vi "_Read.vi"(8 "error in (no error)":errorcluster, 11 "Readable in":refnum<class "Readable.lvclass">) -> (0 "error out":errorcluster, 2 "Data Points":T1, 3 "Readable out":refnum<class "Readable.lvclass">)   [LabVIEW 2009, in "Readable.lvclass"]
doc: "(Protected, Dynamic, Pure Virtual/Abstract) Perform a measurement and return one or more channels of data. Outsiders should not call this method, but instead the public \"Read Data.vi\"."
uses:
  Readable.lvclass
  Data Points.ctl
  Data Point.ctl
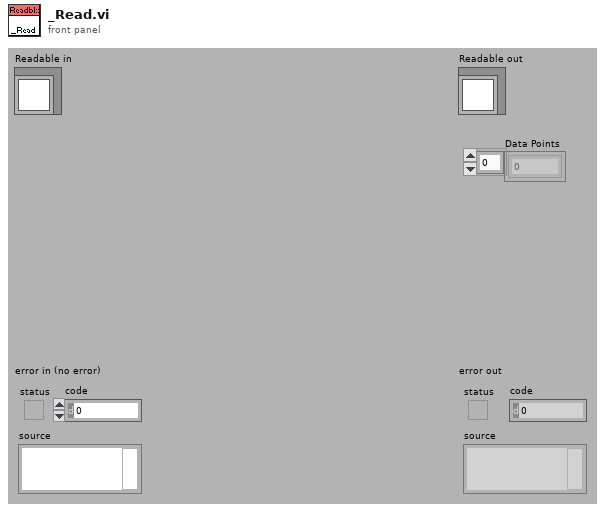
[diagram p1: front panel]
types:
  T1 = typedef "Readable.lvclass/Data Points.ctl" = T2[]
  T2 = typedef "Readable.lvclass/Data Point.ctl" = dbl
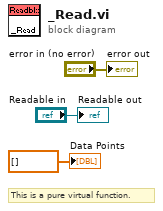
[diagram p0: block diagram]
diagram:
  # "This is a pure virtual function."
  "error out" <- "error in (no error)"
  "Readable out" <- "Readable in"
  "Data Points" <- T1 [] ("Data Points")
